vi "FilterAirmarWind.vi"(9 "Queue timeout (ms)":i32=200, 10 "NotifierReff":T2, 11 "Airmar Wind Queue Cluster":T1) -> ()   [LabVIEW 2013]
doc: "Performs and filtering that we want (default is no filtering) and writes the data to the notifier. If no data is in the queue this VI times out after 'Queue timeout (ms)' has passed and nothing is written to the notifier.\n\nEric Schneider, March 2014"
uses:
  Data/TypeDefs/Notifiers.ctl
  Data/TypeDefs/UTM Location.ctl
  Data/TypeDefs/Sail Set Suggestions.ctl
  Data/TypeDefs/Rudder Set Suggestions.ctl
  Data/TypeDefs/OverrideInformation.ctl
  Data/TypeDefs/OverrideMode.ctl
  Data/TypeDefs/MotorSetup.ctl
  Data/TypeDefs/DynamixelSetupInfo.ctl
  Data/TypeDefs/AirmarStatus.ctl
  Data/TypeDefs/HardwareOnline.ctl
  Data/TypeDefs/DynamixelCycleTracker.ctl
  Data/TypeDefs/RC Input Values.ctl
  Classes/Waypoint/Waypoint.lvclass
  Data/TypeDefs/WindData Queue Cluster.ctl
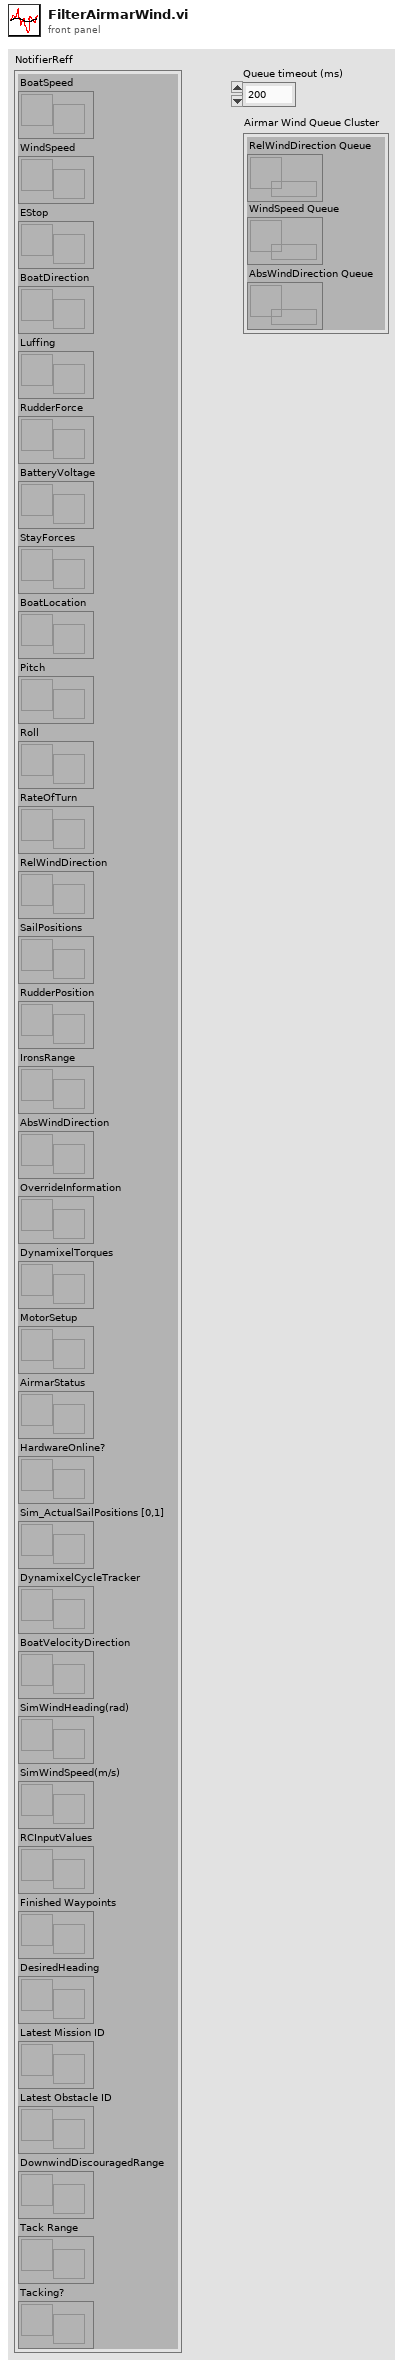
[diagram p1: front panel]
types:
  T1 = typedef "WindData Queue Cluster.ctl" = cluster{"RelWindDirection Queue":refnum<queue>, "WindSpeed Queue":refnum<queue>, "AbsWindDirection Queue":refnum<queue>}
  T2 = typedef "Notifiers.ctl" = cluster{"BoatSpeed":refnum<notifier>, "WindSpeed":refnum<notifier>, "EStop":refnum<notifier>, "BoatDirection":refnum<notifier>, "Luffing":refnum<notifier>, "RudderForce":refnum<notifier>, "BatteryVoltage":refnum<notifier>, "StayForces":refnum<notifier>, "BoatLocation":refnum<notifier>, "Pitch":refnum<notifier>, "Roll":refnum<notifier>, "RateOfTurn":refnum<notifier>, "RelWindDirection":refnum<notifier>, "SailPositions":refnum<notifier>, "RudderPosition":refnum<notifier>, "IronsRange":refnum<notifier>, "AbsWindDirection":refnum<notifier>, "OverrideInformation":refnum<notifier>, "DynamixelTorques":refnum<notifier>, "MotorSetup":refnum<notifier>, "AirmarStatus":refnum<notifier>, "HardwareOnline?":refnum<notifier>, "Sim_ActualSailPositions [0,1]":refnum<notifier>, "DynamixelCycleTracker":refnum<notifier>, "BoatVelocityDirection":refnum<notifier>, "SimWindHeading(rad)":refnum<notifier>, "SimWindSpeed(m/s)":refnum<notifier>, "RCInputValues":refnum<notifier>, "Finished Waypoints":refnum<notifier>, "DesiredHeading":refnum<notifier>, "Latest Mission ID":refnum<notifier>, "Latest Obstacle ID":refnum<notifier>, "DownwindDiscouragedRange":refnum<notifier>, "Tack Range":refnum<notifier>, "Tacking?":refnum<notifier>}
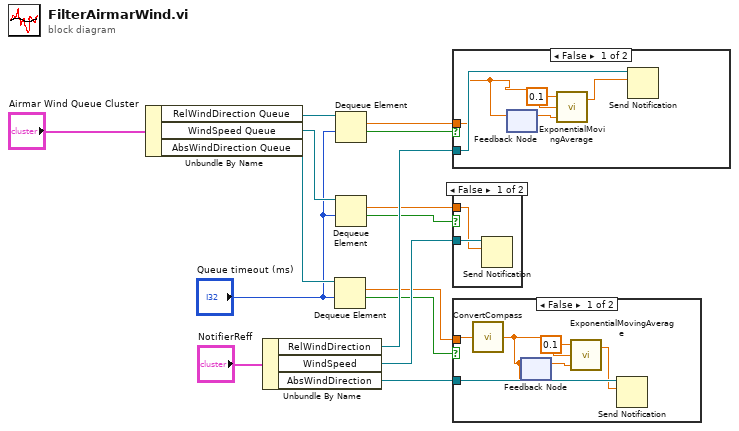
[diagram p0: block diagram]
diagram:
  n1 = Unbundle By Name("Airmar Wind Queue Cluster") -> ("RelWindDirection Queue"=w12:refnum<queue>, "WindSpeed Queue"=w10:refnum<queue>, "AbsWindDirection Queue"=w4:refnum<queue>)
  n2 = Unbundle By Name("NotifierReff") -> ("RelWindDirection"=w11:refnum<notifier>, "WindSpeed"=w9:refnum<notifier>, "AbsWindDirection"=w5:refnum<notifier>)
  n3 = Dequeue Element(queue=w4, timeout in ms (-1)="Queue timeout (ms)") -> (element=w1:dbl, timed out?=w2:bool)  [unwired: 1 in, 2 out]
  n4 = Dequeue Element(queue=w12, timeout in ms (-1)="Queue timeout (ms)") -> (element=w15:dbl, timed out?=w6:bool)  [unwired: 1 in, 2 out]
  n5 = Dequeue Element(queue=w10, timeout in ms (-1)="Queue timeout (ms)") -> (element=w8:dbl, timed out?=w7:bool)  [unwired: 1 in, 2 out]
  n6 = case shown="False" w6 {
    tunnel: w15 -> [w17 _]
    tunnel: w11 -> [w20 _]
    frame False {
      n7 = feedback #1() -> (w19:dbl)  [unwired: 1 in]
      n8 = feedback-in #1(w17) -> ()
      n9 = call "ExponentialMovingAverage.vi"("old value"=w19, "current value"=w17, "weight"=0.1) -> ("average"=w16:dbl)  [unwired: 1 in]
      n10 = Send Notification(notification=w16, notifier=w20) -> ()  [unwired: 1 in, 2 out]
    }
    frame True {
    }
  }
  n11 = case shown="False" w7 {
    tunnel: w9 -> [w22 _]
    tunnel: w8 -> [w21 _]
    frame False {
      n12 = Send Notification(notification=w21, notifier=w22) -> ()  [unwired: 1 in, 2 out]
    }
    frame True {
    }
  }
  n13 = case shown="False" w2 {
    tunnel: w5 -> [w28 _]
    tunnel: w1 -> [w27 _]
    frame False {
      n14 = call "ConvertCompass.vi"("Numeric"=w27) -> ("Heading from East"=w24:dbl)
      n15 = feedback-in #2(w24) -> ()
      n16 = feedback #2(w24) -> (w25:dbl)
      n17 = call "ExponentialMovingAverage.vi"("old value"=w25, "current value"=w24, "weight"=0.1) -> ("average"=w26:dbl)  [unwired: 1 in]
      n18 = Send Notification(notification=w26, notifier=w28) -> ()  [unwired: 1 in, 2 out]
    }
    frame True {
    }
  }
